vi "DigitalOutputClose.vi"(8 "error in":errorcluster, 11 "Device In":u64) -> (0 "error out":errorcluster)   [LabVIEW 2012, in "Phidget Digital Output.lvlib"]
doc: "${DigitalOutput:CloseHeader}"
uses:
  <instrlib>/Phidgets/Phidget Digital Output/Phidget Digital Output.lvlib
  <instrlib>/Phidgets/Phidget Common/Phidget Common.lvlib
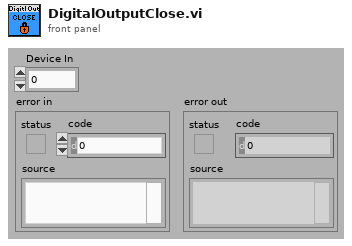
[diagram p1: front panel]
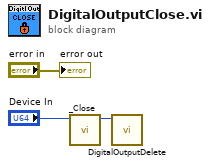
[diagram p0: block diagram]
diagram:
  n1 = call <instrlib>:"_Close.vi"("Device In"="Device In") -> ("Device Out"=w1:u64)  [unwired: 9 in, 1 out]
  n2 = call <instrlib>:"DigitalOutputDelete.vi"("Device In"=w1) -> ()  [unwired: 10 in, 1 out]
  "error out" <- "error in"
